vi "JLINKARM Set Speed.vi"(8 "error in (no error)":errorcluster, 11 "Speed":u32) -> (0 "error out":errorcluster)   [LabVIEW 2020, in "JLinkARM.lvlib"]
doc: "JLINKARMDLL_API void JLINKARM_SetSpeed (U32 Speed);"
uses:
  Lib/JLinkARM.lvlib
  JLinkARM.dll
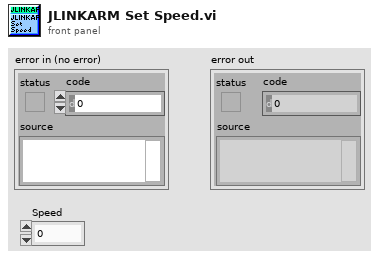
[diagram p1: front panel]
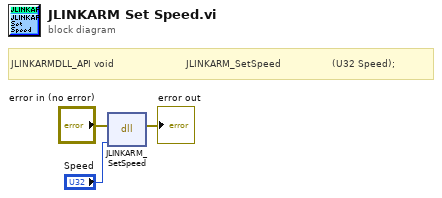
[diagram p0: block diagram]
diagram:
  # "JLINKARMDLL_API void                        JLINKARM_SetSpeed                 (U32 Speed);"
  n1 = dll-call lib="C:/Users/anybody/Desktop/JLinkARM.*" fn="JLINKARM_SetSpeed"(error in="error in (no error)", "Speed"="Speed") -> (error out=→"error out":errorcluster)  [unwired: 4 in, 1 out]
